vi "Configure Calc Null.vi"(7 "NULL Constant (0.0)":dbl min=-999999000000.0 max=999999000000.0 step=1e-14 format="%_6g", 8 "error in (no error)":errorcluster, 9 "Null (0: Off)":u16(ring) format="%_1g" items=["Off", "On"], 10 "Enable NULL Constant (F: Disable)":bool, 11 "VISA resource name":refnum<visa-resource-name>) -> (0 "error out":errorcluster, 3 "VISA resource name out":refnum<visa-resource-name>)   [LabVIEW 2017, in "ADCMT7451_ADC.lvlib"]
doc: "Enables or disables Null calculation."
uses:
  ADCMT7451_ADC.lvlib
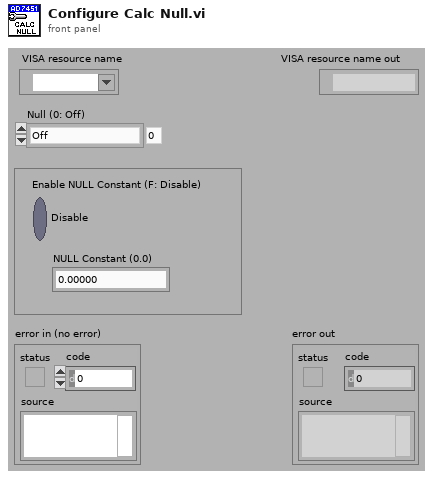
[diagram p1: front panel]
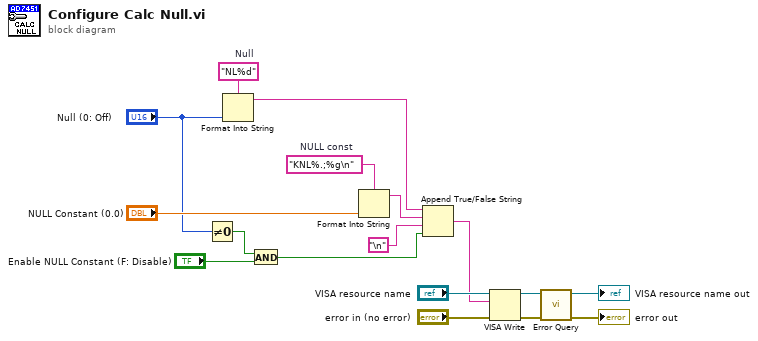
[diagram p0: block diagram]
diagram:
  w3 = "NL%d"  # Null
  w11 = "KNL%.;%g\n"  # NULL const
  n1 = Not Equal To 0?(x="Null (0: Off)") -> (x != 0?=w5:bool)
  n2 = Format Into String(format string=w3, "Null (0: Off)") -> (resulting string=w1:string)  [unwired: 2 in, 1 out]
  n3 = And(x=w5, y="Enable NULL Constant (F: Disable)") -> (x .and. y?=w4:bool)
  n4 = Format Into String(format string=w11, "NULL Constant (0.0)") -> (resulting string=w9:string)  [unwired: 2 in, 1 out]
  n5 = Append True/False String(1:w4, 2:"\n", 3:w9, 4:w1) -> (0:w7:string)
  n6 = VISA Write(VISA resource name="VISA resource name", write buffer=w7, error in (no error)="error in (no error)") -> (VISA resource name out=w13:refnum<visa-resource-name>, error out=w12:errorcluster)  [unwired: 1 out]
  n7 = call "Error Query.vi"("error in (no error)"=w12, "VISA resource name"=w13) -> ("error out"=→"error out":errorcluster, "VISA resource name out"=→"VISA resource name out":refnum<visa-resource-name>)  [unwired: 6 in, 2 out]
